vi "MPM_Get_LAN_PortNumber.vi"(8 "error in (no error)":errorcluster, 11 ".NET Reference in":refnum<k24>) -> (0 "error out":errorcluster, 2 "port out":i32, 3 "Reference out":refnum<k24>)   [LabVIEW 2017]
uses:
  LV_IL_Sample/DLL/InstrumentDLL.dll
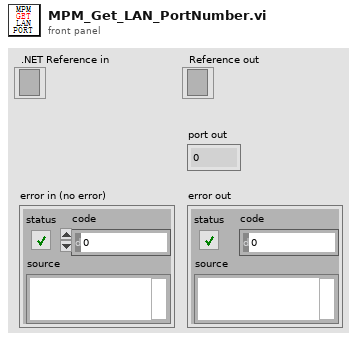
[diagram p1: front panel]
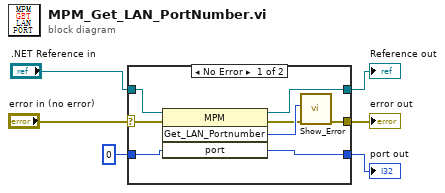
[diagram p0: block diagram]
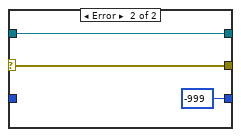
[diagram p2: hidden frame]
diagram:
  n1 = case shown="No Error" "error in (no error)" {
    selector: "error in (no error)" -> [w10 w17]
    tunnel: [w14 -999 ("port")] -> w6
    tunnel: ".NET Reference in" -> [w13 w16]
    tunnel: [w12 w16] -> w4
    tunnel: 0 ("port") -> [w11 _]
    tunnel: [w7 w17] -> w1
    frame No Error {
      n2 = invoke class="MPM" method="Get_LAN_Portnumber"(reference=w13, error in=w10, "port"=w11) -> (reference out=w12:refnum<k24>, error out=w8:errorcluster, "Get_LAN_Portnumber"=w9:i32, "port"=w14:i32)  [unwired: 1 in]
      n3 = call "Show_Error.vi"("error in (no error)"=w8, "Error"=w9) -> ("error out"=w7:errorcluster)  [unwired: 9 in]
    }
    frame Error {
    }
  }
  "port out" <- w6
  "Reference out" <- w4
  "error out" <- w1
